vi "Percent-Encode Path.vi"(10 "Path":string) -> (2 "Pct-Encoded Path":string)   [LabVIEW 2013, in "openURI.lvlib" / "URI-Component.Path.lvclass"]
uses:
  URI-Component.Path.lvclass
  openURI.lvlib
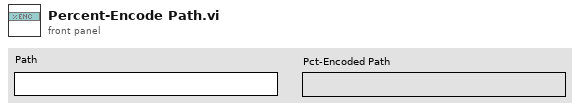
[diagram p1: front panel]
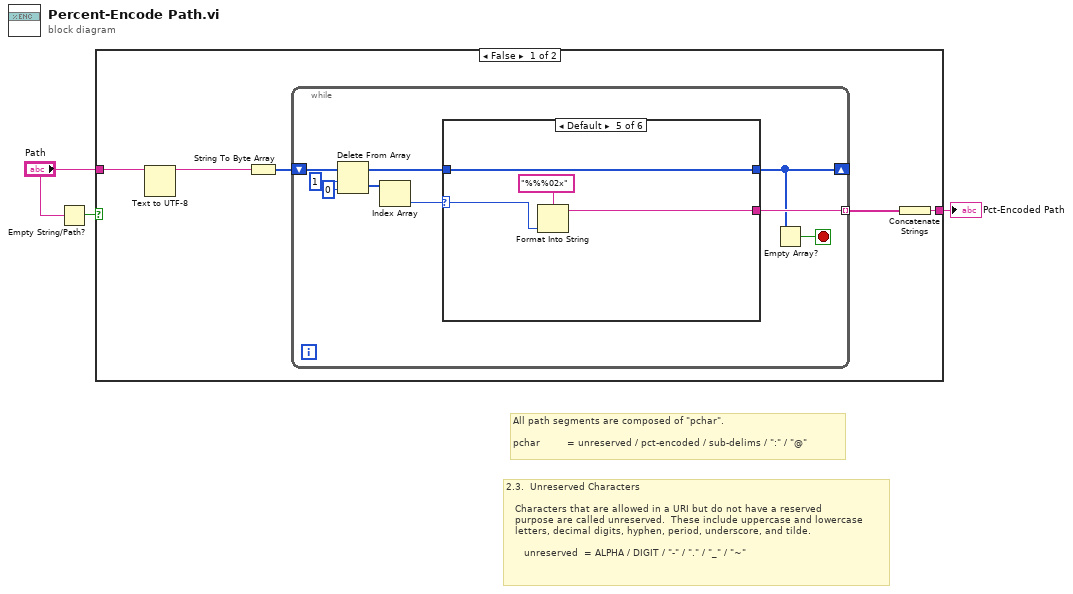
[diagram p0: block diagram]
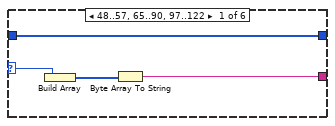
[diagram p2: hidden frame]
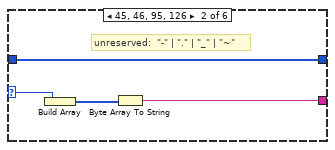
[diagram p3: hidden frame]
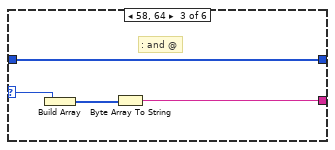
[diagram p4: hidden frame]
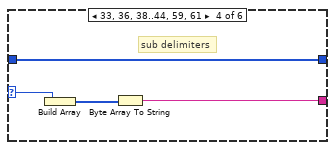
[diagram p5: hidden frame]
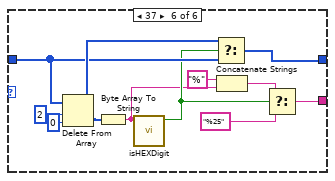
[diagram p6: hidden frame]
diagram:
  # "2.3.  Unreserved Characters\n\n   Characters that are allowed in a URI but do not have a reserved\n   purpose are called unreserved.  These include uppercase and lowercase\n   letters, decimal digits, hyphen, period, underscore, and tilde.\n\n      unreserved  = ALPHA / DIGIT / \"-\" / \".\" / \"_\" / \"~\""
  # "All path segments are composed of \"pchar\".\n\npchar         = unreserved / pct-encoded / sub-delims / \":\" / \"@\""
  n1 = Empty String/Path?(string/path="Path") -> (empty?=w2:bool)
  n2 = case shown="False" w2 {
    tunnel: "Path" -> [w5 _]
    tunnel: [w6 _] -> w3
    frame False {
      n3 = Text to UTF-8(11:w5) -> (3:w4:string)  [unwired: 1 in, 1 out]
      n4 = String To Byte Array(string=w4) -> (unsigned byte array=w8:u8[])
      n5 = while {
        tunnel: [w17] -> w7 mode=indexing
        shift-right: [w10] -> _
        shift-left: w8 -> [w16]
        stop <- w9 stop-if-true
        n6 = Delete From Array(array=w16, length=1, index=0) -> (deleted portion=w13:u8[], array with subset deleted=w11:u8[])
        n7 = Index Array(array=w13) -> (element=w12:u8)  [unwired: 1 in]
        n8 = case shown="Default" w12 {
          selector: w12 -> [w21 w25 w29 w33 w37 _]
          tunnel: [w19 w23 w27 w31 w35 w42] -> w17
          tunnel: w11 -> [w18 w22 w26 w30 w34 w45]
          tunnel: [w18 w22 w26 w30 w34 w44] -> w10
          frame 48..57, 65..90, 97..122 {
            n9 = Build Array(w21) -> (w20:u8[])
            n10 = Byte Array To String(unsigned byte array=w20) -> (string=w19:string)
          }
          frame 45, 46, 95, 126 {
            # "unreserved:  \"-\" | \".\" | \"_\" | \"~\""
            n11 = Build Array(w25) -> (w24:u8[])
            n12 = Byte Array To String(unsigned byte array=w24) -> (string=w23:string)
          }
          frame 58, 64 {
            # ": and @"
            n13 = Build Array(w29) -> (w28:u8[])
            n14 = Byte Array To String(unsigned byte array=w28) -> (string=w27:string)
          }
          frame 33, 36, 38..44, 59, 61 {
            # "sub delimiters"
            n15 = Build Array(w33) -> (w32:u8[])
            n16 = Byte Array To String(unsigned byte array=w32) -> (string=w31:string)
          }
          frame Default {
            n17 = Format Into String(format string="%%%02x", w37) -> (resulting string=w35:string)  [unwired: 2 in, 1 out]
          }
          frame 37 {
            n18 = Delete From Array(array=w45, length=2, index=0) -> (deleted portion=w47:u8[], array with subset deleted=w46:u8[])
            n19 = Byte Array To String(unsigned byte array=w47) -> (string=w40:string)
            n20 = call "isHEXDigit.vi"("characters"=w40) -> ("HEX Digits"=w43:bool)  [unwired: 10 in]
            n21 = Select(t=w46, s=w43, f=w45) -> (s? t:f=w44:u8[])
            n22 = Concatenate Strings("%" ("string"), w40) -> (w39:string)
            n23 = Select(t=w39, s=w43, f="%25" ("string")) -> (s? t:f=w42:string)
          }
        }
        n24 = Empty Array?(array=w10) -> (empty?=w9:bool)
      }
      n25 = Concatenate Strings(w7) -> (w6:string)
    }
    frame True {
    }
  }
  "Pct-Encoded Path" <- w3
